vi "Set_right_exp.vi"(8 "error in (no error)":errorcluster, 10 "Experiment in":refnum<class "Experiment.lvclass">, 11 "Control-Client in":refnum<class "Control-Client.lvclass">) -> (0 "error out":errorcluster, 3 "Control-Client out":refnum<class "Control-Client.lvclass">)   [LabVIEW 2020, in "Control-Client.lvclass"]
uses:
  Control-Client.lvclass
  Experiments/Experiment.lvclass
  Control-Client.lvclass/Control-Client.ctl
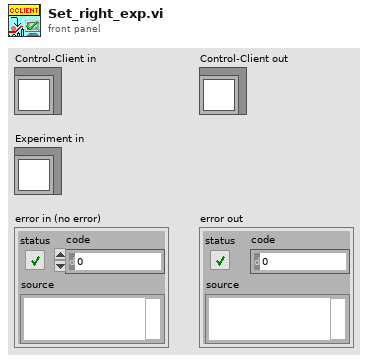
[diagram p1: front panel]
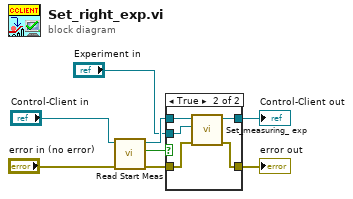
[diagram p0: block diagram]
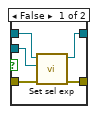
[diagram p2: hidden frame]
diagram:
  n1 = call "Read Start Meas.vi"("error in (no error)"="error in (no error)", "Control-Client in"="Control-Client in") -> ("error out"=w7:errorcluster, "Start Meas"=w8:bool, "Control-Client out"=w6:refnum<class "Control-Client.lvclass">)  [unwired: 7 in]
  n2 = case shown="True" w8 {
    tunnel: w7 -> [w13 w16]
    tunnel: "Experiment in" -> [w12 w18]
    tunnel: [w11 w14] -> w2
    tunnel: [w10 w15] -> w3
    tunnel: w6 -> [w9 w17]
    frame False {
      n3 = call "Set sel exp.vi"("error in (no error)"=w13, "Experiment"=w12, "Control-Client in"=w9) -> ("error out"=w10:errorcluster, "Control-Client out"=w11:refnum<class "Control-Client.lvclass">)  [unwired: 7 in]
    }
    frame True {
      n4 = call "Set_measuring_ exp.vi"("error in (no error)"=w16, "Experiment"=w18, "Control-Client in"=w17) -> ("error out"=w15:errorcluster, "Control-Client out"=w14:refnum<class "Control-Client.lvclass">)  [unwired: 7 in]
    }
  }
  "error out" <- w3
  "Control-Client out" <- w2
